vi "Load Hardware.vi"(8 "error in (no error)":errorcluster, 10 "Program only changes":bool=TRUE, 11 "TestMenu in":refnum<class "TestMenu.lvclass">) -> (0 "error out":errorcluster, 3 "TestMenu out":refnum<class "TestMenu.lvclass">)   [LabVIEW 2013, in "TestMenu.lvclass"]
uses:
  TestMenu.lvclass
  Device/Device.lvclass
panel:
  # "encapsulate HWI in cluser so each \"last encountered\"\ncan be a different length."
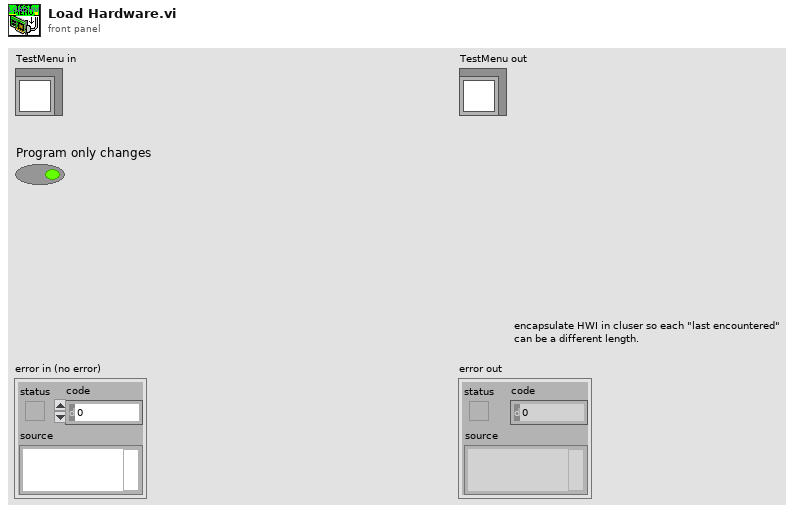
[diagram p1: front panel]
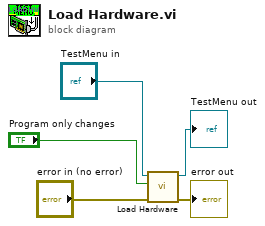
[diagram p0: block diagram]
diagram:
  n1 = call-parent "Load Hardware.vi"("error in (no error)"="error in (no error)", "Program only changes"="Program only changes", "Device in"="TestMenu in") -> ("error out"=→"error out":errorcluster, "Device out"=→"TestMenu out":refnum<class "TestMenu.lvclass">)  [unwired: 7 in]
